vi "Load Settings from XML.vi"(8 "error in (no error)":errorcluster, 11 "Settings in":T1={"Hardware Configuration"={"VISA resource name"="", "Mode (0: Normal) "=0, "Voltage"={"Element (0: All)"=0, "V Range (200)"=4}, "Current"={"A Range (2)"=7, "A Terminal (0: 5A)"=0, "Element (0: ALL)"=0}, "Observation Time"=10, "Modules on/off"={"Module 1"=FALSE, "Module 2"=FALSE, "Module 3"=FALSE, "Module 4"=FALSE}}, "Logging Configuration"={"Log File Base Path"=path "", "TDMS File Reference"=refnum, "Naked Sphere Module"=1, "Insulated Sphere Module"=2}} {"Logging Configuration"."Insulated Sphere Module" min=1 max=4 step=1; "Logging Configuration"."Naked Sphere Module" min=1 max=4 step=1; "Hardware Configuration"."Observation Time" items=["1ksec", "400sec", "200sec", "100sec", "40sec", "20sec", "10sec", "4sec", "2sec", "1sec", "400msec", "200msec", "100msec", "40msec", "20msec", "10msec", "4msec", "2msec", "1msec", "400usec", "200usec", "100usec", "40usec", "20usec", "10usec"]; "Hardware Configuration"."Mode (0: Normal)" items=["Normal", "Harmonics"]; "Hardware Configuration"."Current"."Element (0: ALL)" items=["All", "Element 1", "Element 2", "Element 3", "Element 4"]; "Hardware Configuration"."Current"."A Terminal (0: 5A)" items=["5A", "20A", "Sensor"]; "Hardware Configuration"."Current"."A Range (2)" items=["AUTO", "0.1", "0.2", "0.4", "1", "2", "4", "10", "20", "40", "100"]; "Hardware Configuration"."Voltage"."V Range (200)" items=["AUTO", "30", "60", "120", "200", "300", "600", "1200", "2000"]; "Hardware Configuration"."Voltage"."Element (0: All)" items=["All", "Element 1", "Element 2", "Element 3", "Element 4"]}) -> (0 "error out":errorcluster, 3 "Settings out":T1={"Hardware Configuration"={"VISA resource name"="", "Mode (0: Normal) "=0, "Voltage"={"Element (0: All)"=0, "V Range (200)"=4}, "Current"={"A Range (2)"=7, "A Terminal (0: 5A)"=0, "Element (0: ALL)"=0}, "Observation Time"=10, "Modules on/off"={"Module 1"=FALSE, "Module 2"=FALSE, "Module 3"=FALSE, "Module 4"=FALSE}}, "Logging Configuration"={"Log File Base Path"=path "", "TDMS File Reference"=refnum, "Naked Sphere Module"=1, "Insulated Sphere Module"=2}} {"Logging Configuration"."Insulated Sphere Module" min=1 max=4 step=1; "Logging Configuration"."Naked Sphere Module" min=1 max=4 step=1; "Hardware Configuration"."Observation Time" items=["1ksec", "400sec", "200sec", "100sec", "40sec", "20sec", "10sec", "4sec", "2sec", "1sec", "400msec", "200msec", "100msec", "40msec", "20msec", "10msec", "4msec", "2msec", "1msec", "400usec", "200usec", "100usec", "40usec", "20usec", "10usec"]; "Hardware Configuration"."Mode (0: Normal)" items=["Normal", "Harmonics"]; "Hardware Configuration"."Current"."Element (0: ALL)" items=["All", "Element 1", "Element 2", "Element 3", "Element 4"]; "Hardware Configuration"."Current"."A Terminal (0: 5A)" items=["5A", "20A", "Sensor"]; "Hardware Configuration"."Current"."A Range (2)" items=["AUTO", "0.1", "0.2", "0.4", "1", "2", "4", "10", "20", "40", "100"]; "Hardware Configuration"."Voltage"."V Range (200)" items=["AUTO", "30", "60", "120", "200", "300", "600", "1200", "2000"]; "Hardware Configuration"."Voltage"."Element (0: All)" items=["All", "Element 1", "Element 2", "Element 3", "Element 4"]})   [LabVIEW 2013, in "Yokogawa.lvlib" / "YKPZ400 Settings.lvlib"]
doc: "Attempts to load previous user specified settings from an XML file.\n\nThis VI will not generate an error. If a suitable XML file can't be loaded and parsed then it will simply return the default settings."
uses:
  YKPZ400 Settings.lvlib
  Settings.ctl
  Acquisition/Hardware Configuration.ctl
  Logging/Logging Configuration.ctl
  <vilib>/Utility/xml.llb/Read From XML File(string).vi
  <vilib>/Utility/xml.llb/Write to XML File(string).vi
  Acquisition/YKPZ400 Acquisition.lvlib
  Logging/YKPZ400 Logging.lvlib
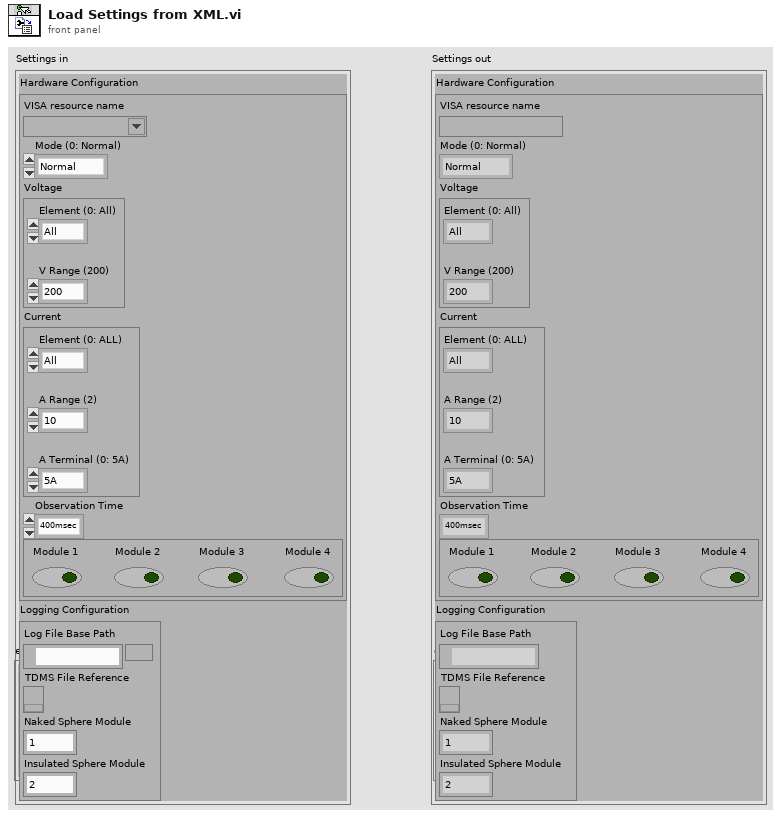
[diagram p1: front panel]
types:
  T1 = typedef "Yokogawa.lvlib/YKPZ400 Settings.lvlib/Settings.ctl" = cluster{"Hardware Configuration":T2, "Logging Configuration":T3}
  T2 = typedef "Yokogawa.lvlib/YKPZ400 Acquisition.lvlib/Hardware Configuration.ctl" = cluster{"VISA resource name":refnum<visa-resource-name>, "Mode (0: Normal) ":u16, "Voltage":cluster{"Element (0: All)":u16, "V Range (200)":u16}, "Current":cluster{"A Range (2)":u16, "A Terminal (0: 5A)":u16, "Element (0: ALL)":u16}, "Observation Time":u16, "Modules on/off":cluster{"Module 1":bool, "Module 2":bool, "Module 3":bool, "Module 4":bool}}
  T3 = typedef "Yokogawa.lvlib/YKPZ400 Logging.lvlib/Logging Configuration.ctl" = cluster{"Log File Base Path":path, "TDMS File Reference":refnum<k34>, "Naked Sphere Module":i32, "Insulated Sphere Module":i32}
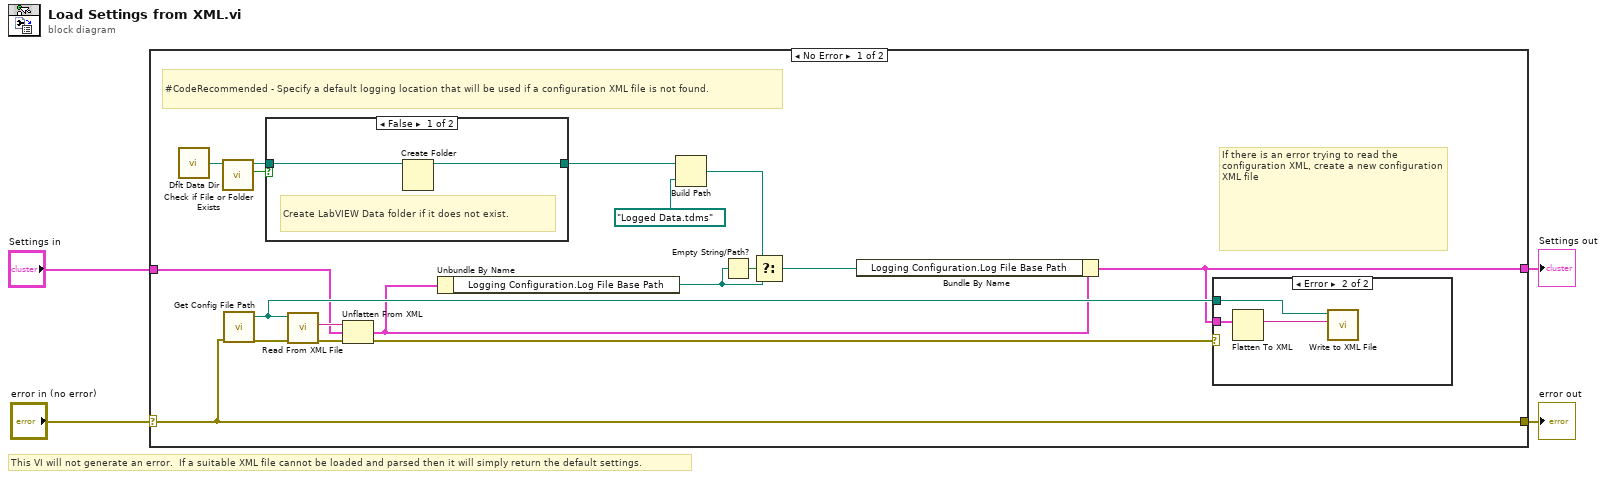
[diagram p0: block diagram]
diagram:
  # "This VI will not generate an error.  If a suitable XML file cannot be loaded and parsed then it will simply return the default settings."
  n1 = case shown="No Error" "error in (no error)" {
    selector: "error in (no error)" -> [w20 w30]
    tunnel: [w20 w30] -> w3
    tunnel: "Settings in" -> [w15 w29]
    tunnel: [w9 w29] -> w1
    frame No Error {
      # "If there is an error trying to read the configuration XML, create a new configuration XML file"
      # "#CodeRecommended - Specify a default logging location that will be used if a configuration XML file is not found."
      n2 = call <vilib>:"Dflt Data Dir.vi"() -> ("App:Default Data Directory"=w8:path)
      n3 = call <vilib>:"Check if File or Folder Exists.vi"("path"=w8) -> ("file or folder exists?"=w7:bool, "dup path"=w6:path)  [unwired: 8 in, 1 out]
      n4 = call "Get Config File Path.vi"("error in (no error)"=w20) -> ("error out"=w22:errorcluster, "XML File Path"=w18:path)  [unwired: 9 in]
      n5 = case shown="False" w7 {
        tunnel: w6 -> [w24 w25]
        tunnel: [w23 w25] -> w5
        frame False {
          # "Create LabVIEW Data folder if it does not exist."
          n6 = Create Folder(path (use dialog)=w24) -> (created path=w23:path)  [unwired: 2 in, 2 out]
        }
        frame True {
        }
      }
      n7 = call-poly <vilib>:"Read From XML File.vi"("error in (no error)"=w22, "XML File Path"=w18) -> ("error out"=w17:errorcluster, "XML Elements"=w21:string)  [unwired: 7 in, 1 out]
      n8 = Unflatten From XML(xml string=w21, type=w15, error in (no error)=w17) -> (value=w11:T1, error out=w16:errorcluster)
      n9 = Unbundle By Name(w11) -> ("Logging Configuration.Log File Base Path"=w13:path)
      n10 = Build Path(base path=w5, name or relative path=path "Logged Data.tdms" ("App:Default Data Directory")) -> (appended path=w12:path)
      n11 = Empty String/Path?(string/path=w13) -> (empty?=w14:bool)
      n12 = Select(t=w12, s=w14, f=w13) -> (s? t:f=w10:path)
      n13 = Bundle By Name(cluster=w11, "Logging Configuration.Log File Base Path"=w10) -> (w9:T1)
      n14 = case shown="Error" w16 {
        tunnel: w9 -> [_ w28]
        tunnel: w18 -> [_ w26]
        frame No Error {
        }
        frame Error {
          n15 = Flatten To XML(anything=w28) -> (xml string=w27:string)
          n16 = call-poly <vilib>:"Write to XML File.vi"("XML Input"=w27, "XML File Path"=w26) -> ()  [unwired: 7 in, 3 out]
        }
      }
    }
    frame Error {
    }
  }
  "error out" <- w3
  "Settings out" <- w1
